vi "Page_Advanced_Initialize.vi"(6 "ctl references":T1, 8 "error in (no error)":errorcluster, 11 "AB_EXE in":refnum<class "AB_EXE.lvclass">) -> (0 "error out":errorcluster, 3 "AB_EXE out":refnum<class "AB_EXE.lvclass">)   [LabVIEW 2020, in "AB_EXE.lvclass"]
uses:
  <vilib>/AppBuilder/AB_Classes/EXE/AB_EXE.lvclass
  <resource>/Framework/Providers/Builds/AppBuilder/AB_UI_Page_Advanced_References.ctl
  <resource>/Framework/Providers/Common/provcom_StringGlobals.vi
  <vilib>/AppBuilder/AB_Classes/Application/AB_Application.lvclass
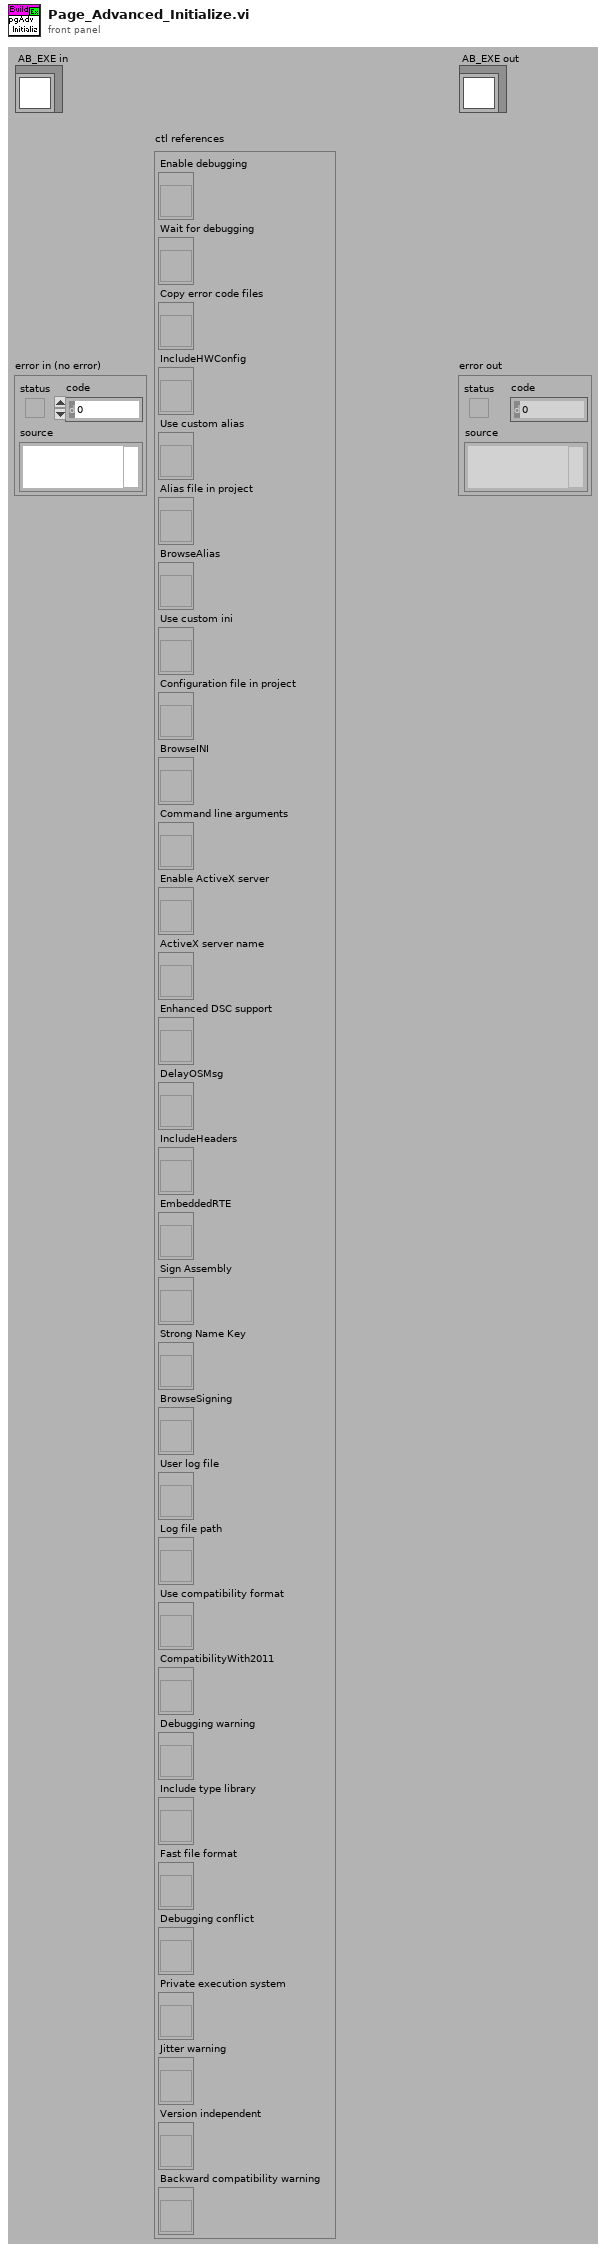
[diagram p1: front panel]
types:
  T1 = typedef "AB_UI_Page_Advanced_References.ctl" = cluster{"Enable debugging":refnum<vi>, "Wait for debugging":refnum<vi>, "Copy error code files":refnum<vi>, "IncludeHWConfig":refnum<vi>, "Use custom alias":refnum<vi>, "Alias file in project":refnum<vi>, "BrowseAlias":refnum<vi>, "Use custom ini":refnum<vi>, "Configuration file in project":refnum<vi>, "BrowseINI":refnum<vi>, "Command line arguments":refnum<vi>, "Enable ActiveX server":refnum<vi>, "ActiveX server name":refnum<vi>, "Enhanced DSC support":refnum<vi>, "DelayOSMsg":refnum<vi>, "IncludeHeaders":refnum<vi>, "EmbeddedRTE":refnum<vi>, "Sign Assembly":refnum<vi>, "Strong Name Key":refnum<vi>, "BrowseSigning":refnum<vi>, "User log file":refnum<vi>, "Log file path":refnum<vi>, "Use compatibility format":refnum<vi>, "CompatibilityWith2011":refnum<vi>, "Debugging warning":refnum<vi>, "Include type library":refnum<vi>, "Fast file format":refnum<vi>, "Debugging conflict":refnum<vi>, "Private execution system":refnum<vi>, "Jitter warning":refnum<vi>, "Version independent":refnum<vi>, "Backward compatibility warning":refnum<vi>}
  T2 = enum32{"invalid OS target", "Mac OS", "Windows 3.1", "Windows 95/NT", "Solaris 1", "Solaris 2", "HP-UX", "PowerMAX", "Linux", "Irix", "Rhapsody", "BeOS", "AIX", "OSF1", "VxWorks", "PharLap", "Carbon", "RTX", "Windows x64", "Linux x64", "Mac OS X x64"}
  T3 = typedef "LVRectTypeDef.ctl" = cluster{"Left":i16, "Top":i16, "Right":i16, "Bottom":i16}
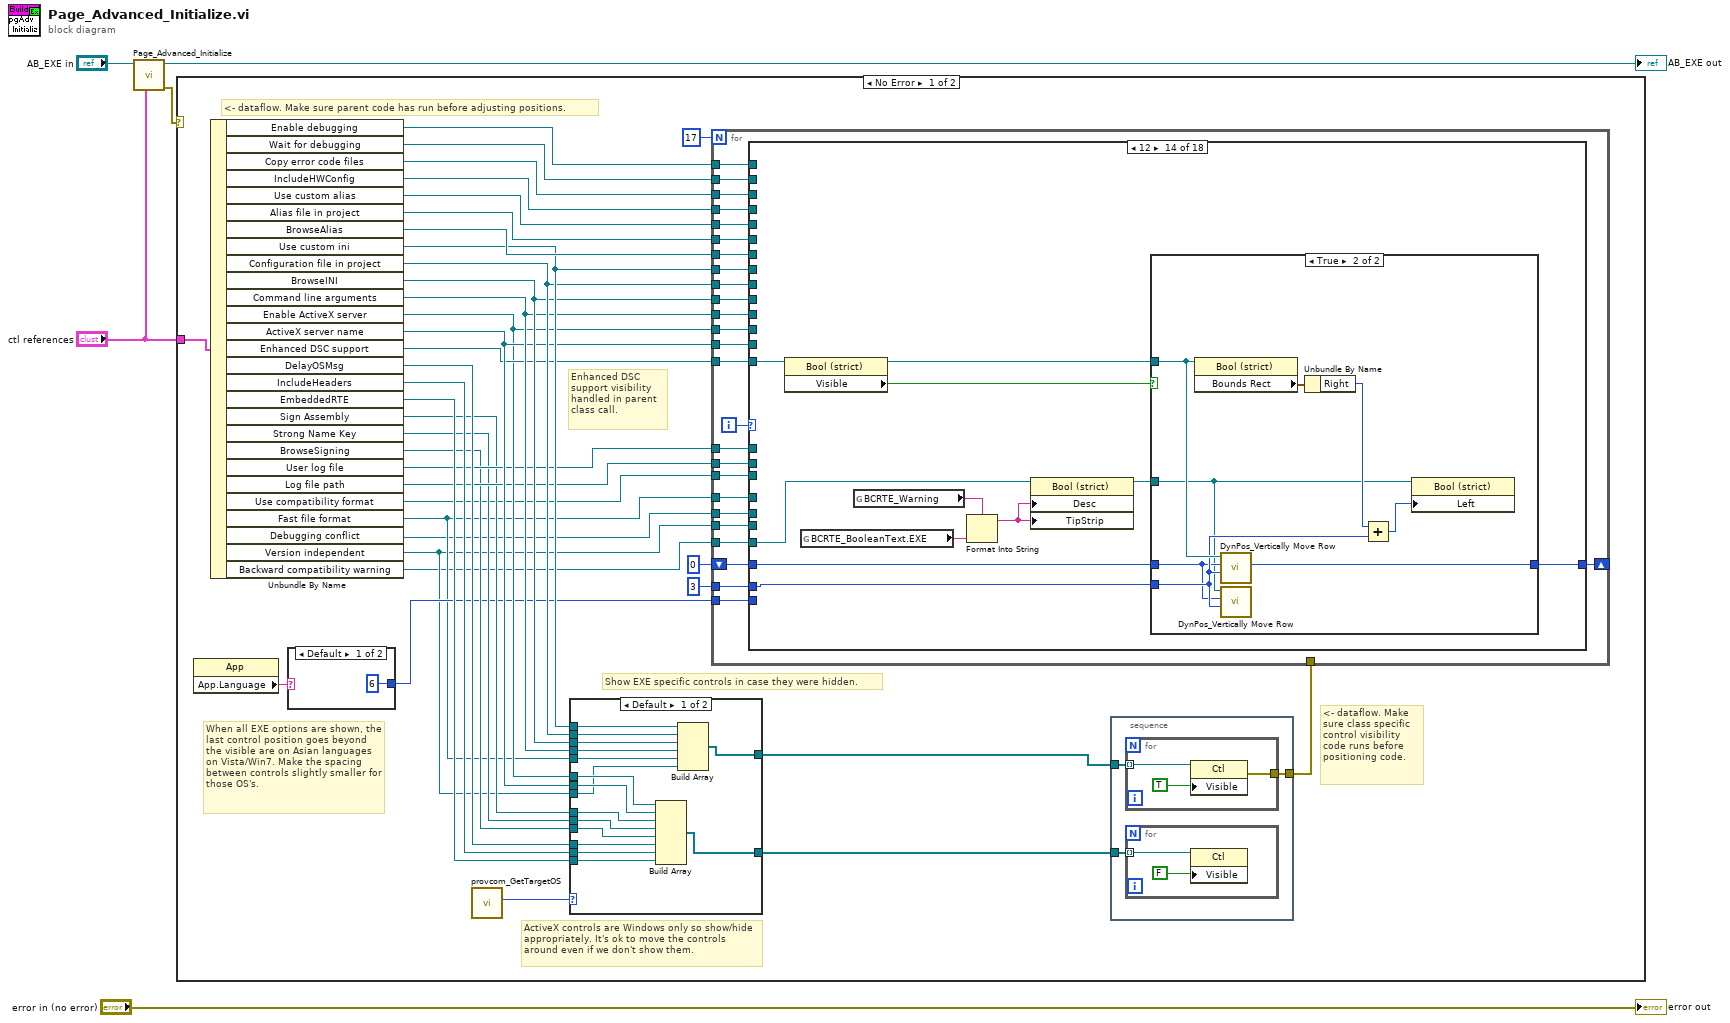
[diagram p0: block diagram]
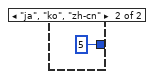
[diagram p2: hidden frame]
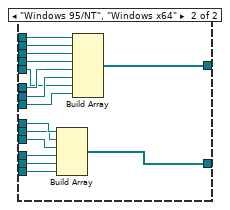
[diagram p3: hidden frame]
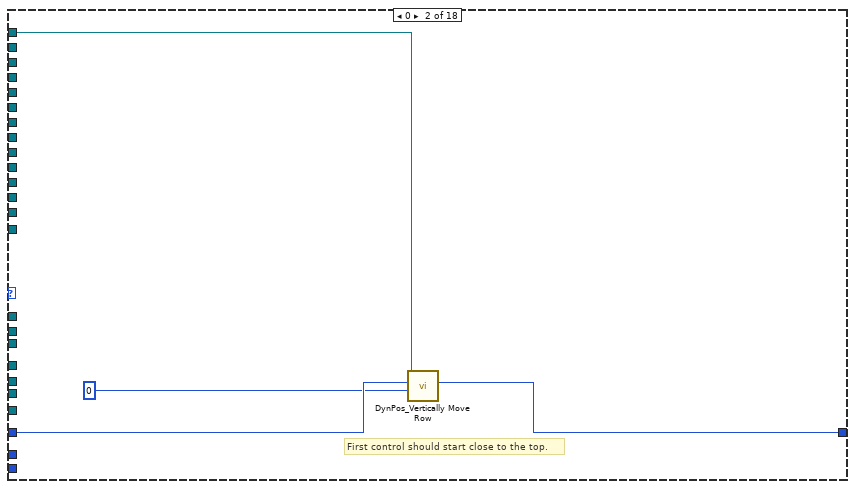
[diagram p5: hidden frame]
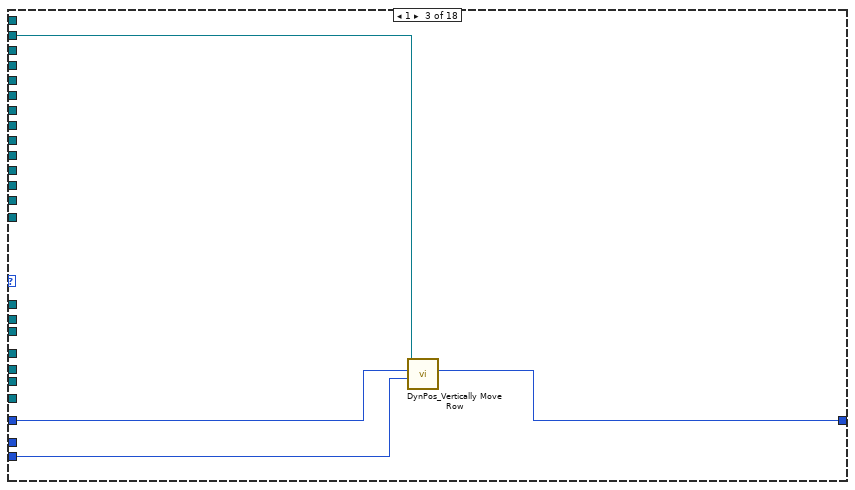
[diagram p6: hidden frame]
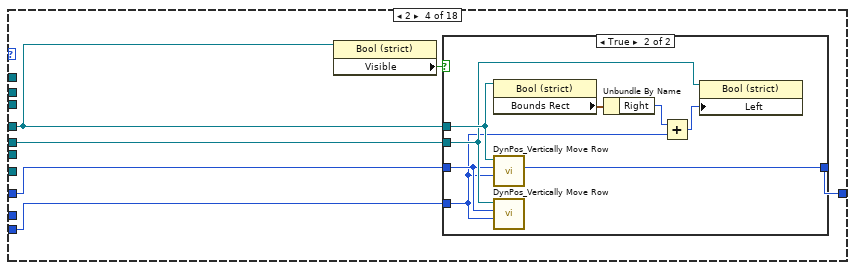
[diagram p7: hidden frame]
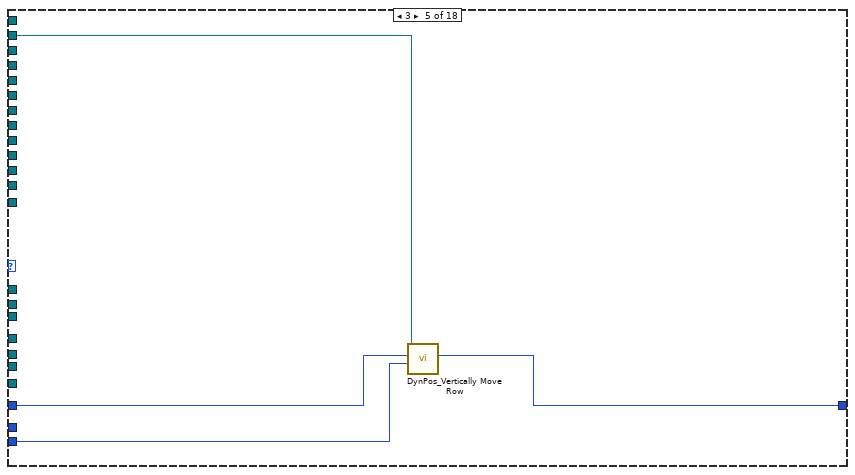
[diagram p9: hidden frame]
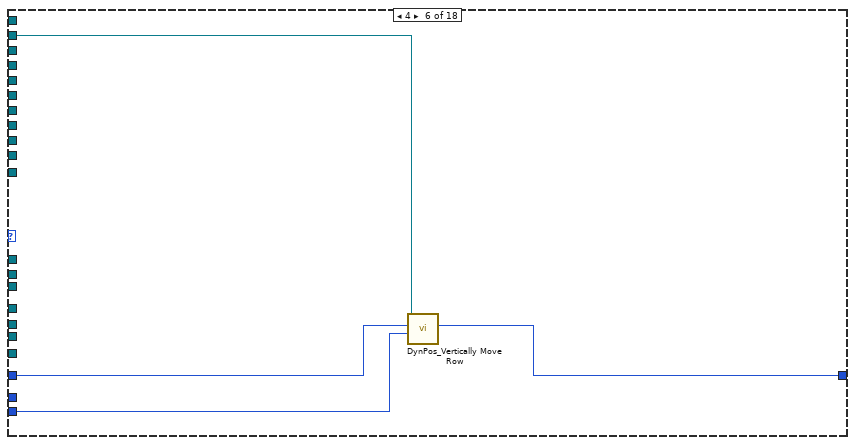
[diagram p10: hidden frame]
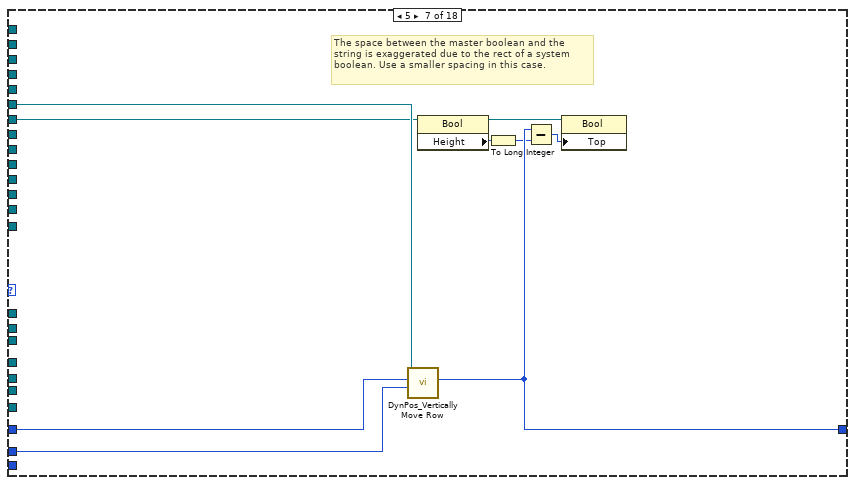
[diagram p11: hidden frame]
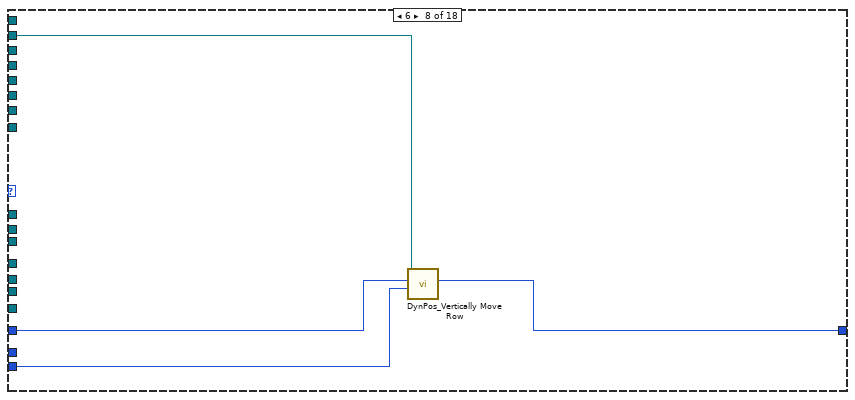
[diagram p12: hidden frame]
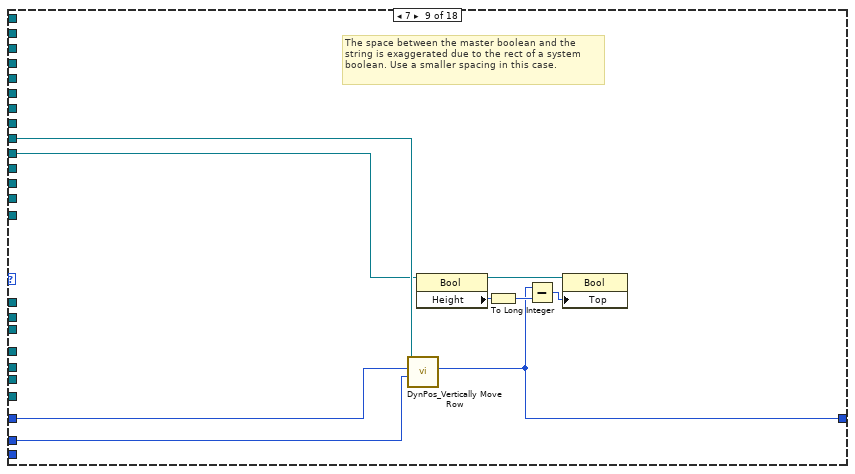
[diagram p13: hidden frame]
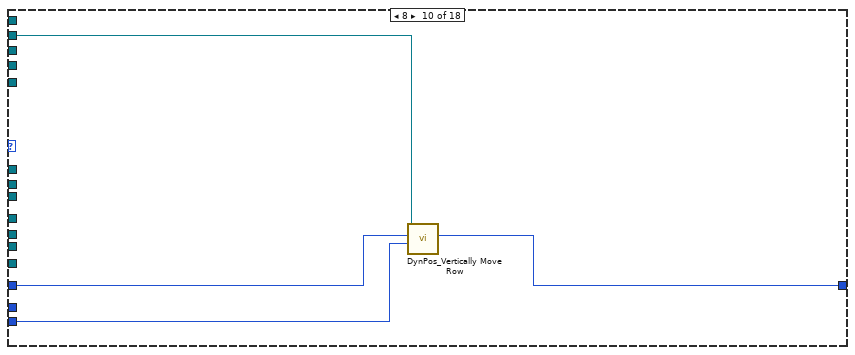
[diagram p14: hidden frame]
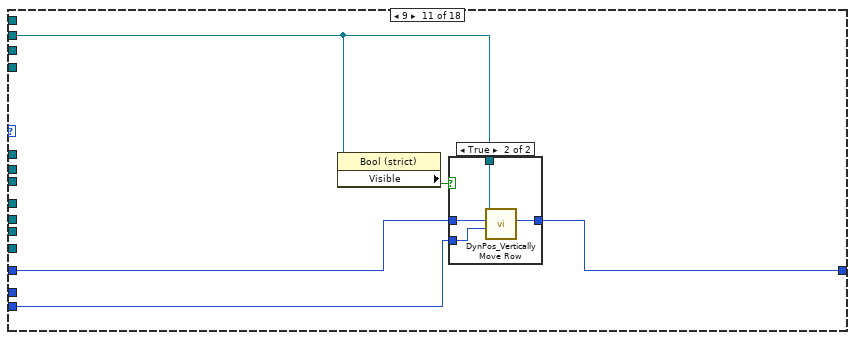
[diagram p15: hidden frame]
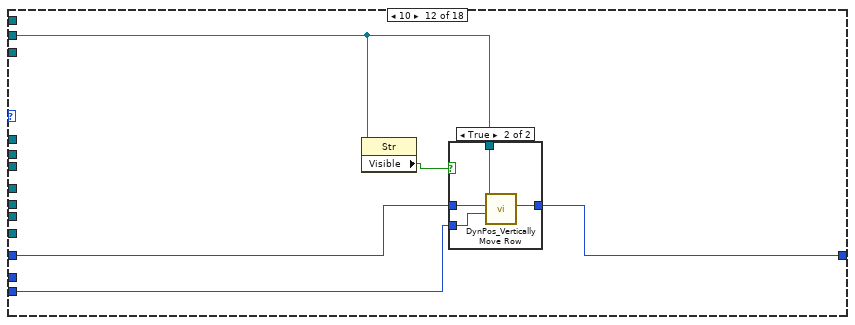
[diagram p17: hidden frame]
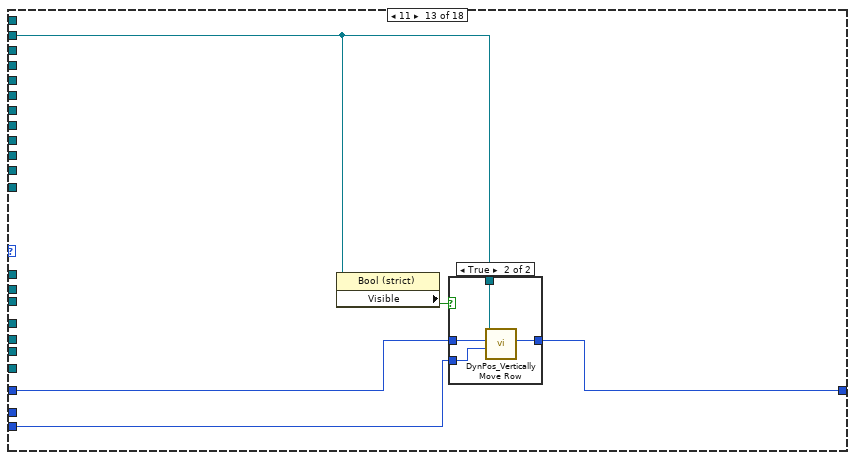
[diagram p19: hidden frame]
diagram:
  n1 = call-parent "Page_Advanced_Initialize.vi"("ctl references"="ctl references", "AB_Application in"="AB_EXE in") -> ("error out"=w1:errorcluster, "AB_Application out"=→"AB_EXE out":refnum<class "AB_EXE.lvclass">)  [unwired: 1 in, 7 out]
  n2 = case shown="No Error" w1 {
    tunnel: "ctl references" -> [w24 _]
    frame No Error {
      # "When all EXE options are shown, the last control position goes beyond the visible are on Asian languages on Vista/Win7. Make the spacing between controls slightly smaller for those OS's."
      # "<- dataflow. Make sure parent code has run before adjusting positions."
      # "<- dataflow. Make sure class specific control visibility code runs before positioning code."
      # "Enhanced DSC support visibility handled in parent class call."
      # "Show EXE specific controls in case they were hidden."
      # "ActiveX controls are Windows only so show/hide appropriately. It's ok to move the controls around even if we don't show them."
      n3 = property class="App"() -> ("App.Language"=w12:string)  [unwired: 2 in, 2 out]
      n4 = Unbundle By Name(w24) -> ("Enable debugging"=w39:refnum<vi>, "Wait for debugging"=w38:refnum<vi>, "Copy error code files"=w37:refnum<vi>, "IncludeHWConfig"=w36:refnum<vi>, "Use custom alias"=w35:refnum<vi>, "Alias file in project"=w34:refnum<vi>, "BrowseAlias"=w33:refnum<vi>, "Use custom ini"=w29:refnum<vi>, "Configuration file in project"=w28:refnum<vi>, "BrowseINI"=w27:refnum<vi>, "Command line arguments"=w26:refnum<vi>, "Enable ActiveX server"=w21:refnum<vi>, "ActiveX server name"=w23:refnum<vi>, "Enhanced DSC support"=w22:refnum<vi>, "DelayOSMsg"=w42:refnum<vi>, "IncludeHeaders"=w41:refnum<vi>, "EmbeddedRTE"=w40:refnum<vi>, "Sign Assembly"=w17:refnum<vi>, "Strong Name Key"=w16:refnum<vi>, "BrowseSigning"=w15:refnum<vi>, "User log file"=w18:refnum<vi>, "Log file path"=w19:refnum<vi>, "Use compatibility format"=w13:refnum<vi>, "Fast file format"=w9:refnum<vi>, "Debugging conflict"=w8:refnum<vi>, "Version independent"=w7:refnum<vi>, "Backward compatibility warning"=w6:refnum<vi>)
      n5 = case shown="Default" w12 {
        tunnel: [6 ("Bottom of last control") 5 ("Bottom of last control")] -> w11
        frame Default {
        }
        frame "ja", "ko", "zh-cn" {
        }
      }
      n6 = call <resource>:"provcom_GetTargetOS.vi"() -> ("App.TargetOS"=w20:T2)  [unwired: 11 out]
      n7 = case shown="Default" w20 {
        tunnel: w42 -> [w66 w84]
        tunnel: w41 -> [w67 w83]
        tunnel: w40 -> [w68 w82]
        tunnel: [w65 w81] -> w30
        tunnel: w23 -> [w58 w75]
        tunnel: w29 -> [w64 w80]
        tunnel: w28 -> [w63 w79]
        tunnel: w27 -> [w62 w78]
        tunnel: w26 -> [w61 w77]
        tunnel: [w60 w76] -> w25
        tunnel: w21 -> [w59 w74]
        tunnel: w17 -> [w57 w73]
        tunnel: w16 -> [w56 w72]
        tunnel: w15 -> [w55 w71]
        tunnel: w9 -> [w54 w70]
        tunnel: w7 -> [w53 w69]
        frame Default {
          n8 = Build Array(w59, w58, w57, w56, w55, w66, w67, w68) -> (w65:refnum<vi>[])
          n9 = Build Array(w64, w63, w62, w61, w54, w53) -> (w60:refnum<vi>[])
        }
        frame "Windows 95/NT", "Windows x64" {
          n10 = Build Array(w73, w72, w71, w84, w83, w82) -> (w81:refnum<vi>[])
          n11 = Build Array(w80, w79, w78, w77, w74, w75, w70, w69) -> (w76:refnum<vi>[])
        }
      }
      n12 = stacked-sequence {
        tunnel: w30 -> [w47]
        tunnel: w25 -> [w46]
        tunnel: [w45] -> w14
        frame #0 {
          n13 = for {
            tunnel: w46 -> [w50] mode=indexing
            tunnel: [w48] -> w45
            n14 = property class="Ctl"(reference=w50, "Visible"=TRUE) -> (error out=w48:errorcluster)  [unwired: 1 in, 1 out]
          }
          n15 = for {
            tunnel: w47 -> [w52] mode=indexing
            n16 = property class="Ctl"(reference=w52, "Visible"=FALSE) -> ()  [unwired: 1 in, 2 out]
          }
        }
      }
      n17 = for {
        N: 17 -> [_]
        tunnel: w39 -> [w109]
        tunnel: w38 -> [w108]
        tunnel: w37 -> [w107]
        tunnel: w36 -> [w106]
        tunnel: w35 -> [w105]
        tunnel: w34 -> [w104]
        tunnel: w33 -> [w103]
        tunnel: w29 -> [w102]
        tunnel: w28 -> [w101]
        shift-right: [w98] -> _
        shift-left: 0 ("Bottom of last control") -> [w100]
        tunnel: w11 -> [w99]
        tunnel: w27 -> [w97]
        tunnel: w26 -> [w96]
        tunnel: w21 -> [w95]
        tunnel: w23 -> [w94]
        tunnel: w22 -> [w93]
        tunnel: w19 -> [w92]
        tunnel: w18 -> [w91]
        tunnel: w14 -> [_]
        tunnel: w13 -> [w90]
        tunnel: 3 ("Bottom of last control") -> [w89]
        tunnel: w9 -> [w88]
        tunnel: w8 -> [w87]
        tunnel: w7 -> [w86]
        tunnel: w6 -> [w85]
        i -> [w110]
        n18 = case shown="12" w110 {
          tunnel: w109 -> [_ w114 _ _ _ _ _ _ _ _ _ _ _ _ _ _ _ _]
          tunnel: w108 -> [_ _ w116 _ _ _ _ _ _ _ _ _ _ _ _ _ _ _]
          tunnel: w107 -> [_ _ _ _ w135 _ _ _ _ _ _ _ _ _ _ _ _ _]
          tunnel: w106 -> [_ _ _ _ _ _ _ _ _ _ _ _ w190 _ _ _ _ _]
          tunnel: w105 -> [_ _ _ _ _ w139 _ _ _ _ _ _ _ _ _ _ _ _]
          tunnel: w104 -> [_ _ _ _ _ _ w150 _ _ _ _ _ _ _ _ _ _ _]
          tunnel: w103 -> [_ _ _ _ _ _ w149 _ _ _ _ _ _ _ _ _ _ _]
          tunnel: w102 -> [_ _ _ _ _ _ _ w152 _ _ _ _ _ _ _ _ _ _]
          tunnel: w101 -> [_ _ _ _ _ _ _ _ w163 _ _ _ _ _ _ _ _ _]
          tunnel: w100 -> [w111 w115 w119 w123 w138 w142 w151 w155 w164 w168 w172 w182 w193 w206 w222 w226 w230 w238]
          tunnel: w99 -> [_ _ w118 w122 w137 w141 _ w154 _ w167 w171 w181 w192 _ w221 w225 w229 w237]
          tunnel: [w111 w113 w117 w125 w136 w140 w145 w153 w158 w166 w170 w180 w191 w209 w220 w224 w228 w236] -> w98
          tunnel: w97 -> [_ _ _ _ _ _ _ _ w159 _ _ _ _ _ _ _ _ _]
          tunnel: w96 -> [_ _ _ _ _ _ _ _ _ w165 _ _ _ _ _ _ _ _]
          tunnel: w95 -> [_ _ _ _ _ _ _ _ _ _ w169 _ _ _ _ _ _ _]
          tunnel: w94 -> [_ _ _ _ _ _ _ _ _ _ _ w179 _ _ _ _ _ _]
          tunnel: w93 -> [_ _ _ _ _ _ _ _ _ _ _ _ _ w204 _ _ _ _]
          tunnel: w92 -> [_ _ _ _ _ _ _ _ _ _ _ _ _ _ _ w223 _ _]
          tunnel: w91 -> [_ _ _ _ _ _ _ _ _ _ _ _ _ _ w219 _ _ _]
          tunnel: w90 -> [_ _ _ _ _ _ _ _ _ _ _ _ _ _ _ _ w227 _]
          tunnel: w89 -> [_ _ _ _ _ _ w143 _ w156 _ _ _ _ w207 _ _ _ _]
          tunnel: w88 -> [_ _ _ w121 _ _ _ _ _ _ _ _ _ _ _ _ _ _]
          tunnel: w87 -> [_ _ _ w124 _ _ _ _ _ _ _ _ _ _ _ _ _ _]
          tunnel: w86 -> [_ _ _ _ _ _ _ _ _ _ _ _ _ _ _ _ _ w234]
          tunnel: w85 -> [_ _ _ _ _ _ _ _ _ _ _ _ _ w203 _ _ _ _]
          frame Default {
          }
          frame 0 {
            # "First control should start close to the top."
            n19 = call <vilib>:"DynPos_Vertically Move Row.vi"("Pixel separation (6)"=0, "Bottom of last control"=w115, "Control"=w114) -> ("Bottom pixel"=w113:i32)  [unwired: 1 in, 7 out]
          }
          frame 1 {
            n20 = call <vilib>:"DynPos_Vertically Move Row.vi"("Pixel separation (6)"=w118, "Bottom of last control"=w119, "Control"=w116) -> ("Bottom pixel"=w117:i32)  [unwired: 1 in, 7 out]
          }
          frame 2 {
            n21 = property class="Bool (strict)"(reference=w121) -> ("Visible"=w120:bool)  [unwired: 1 in, 2 out]
            n22 = case shown="True" w120 {
              tunnel: [w126 w134] -> w125
              tunnel: w121 -> [_ w130]
              tunnel: w124 -> [_ w129]
              tunnel: w123 -> [w126 w128]
              tunnel: w122 -> [_ w127]
              frame False {
              }
              frame True {
                n23 = property class="Bool (strict)"(reference=w130) -> ("Bounds Rect"=w133:T3)  [unwired: 1 in, 2 out]
                n24 = call <vilib>:"DynPos_Vertically Move Row.vi"("Pixel separation (6)"=w127, "Bottom of last control"=w128, "Control"=w130) -> ("Bottom pixel"=w134:i32)  [unwired: 1 in, 7 out]
                n25 = call <vilib>:"DynPos_Vertically Move Row.vi"("Pixel separation (6)"=w127, "Bottom of last control"=w128, "Control"=w129) -> ()  [unwired: 1 in, 8 out]
                n26 = Unbundle By Name(w133) -> ("Right"=w132:i16)
                n27 = Add(x=w132, y=w127) -> (x+y=w131:i32)
                n28 = property class="Bool (strict)"(reference=w129, "Left"=w131) -> ()  [unwired: 1 in, 2 out]
              }
            }
          }
          frame 3 {
            n29 = call <vilib>:"DynPos_Vertically Move Row.vi"("Pixel separation (6)"=w137, "Bottom of last control"=w138, "Control"=w135) -> ("Bottom pixel"=w136:i32)  [unwired: 1 in, 7 out]
          }
          frame 4 {
            n30 = call <vilib>:"DynPos_Vertically Move Row.vi"("Pixel separation (6)"=w141, "Bottom of last control"=w142, "Control"=w139) -> ("Bottom pixel"=w140:i32)  [unwired: 1 in, 7 out]
          }
          frame 5 {
            # "The space between the master boolean and the string is exaggerated due to the rect of a system boolean. Use a smaller spacing in this case."
            n31 = call <vilib>:"DynPos_Vertically Move Row.vi"("Pixel separation (6)"=w143, "Bottom of last control"=w151, "Control"=w150) -> ("Bottom pixel"=w145:i32)  [unwired: 1 in, 7 out]
            n32 = property class="Bool"(reference=w149) -> (reference out=w148:refnum<vi>, "Height"=w147:u32)  [unwired: 1 in, 1 out]
            n33 = To Long Integer(number=w147) -> (32bit integer=w144:i32)
            n34 = Subtract(x=w145, y=w144) -> (x-y=w146:i32)
            n35 = property class="Bool"(reference=w148, "Top"=w146) -> ()  [unwired: 1 in, 2 out]
          }
          frame 6 {
            n36 = call <vilib>:"DynPos_Vertically Move Row.vi"("Pixel separation (6)"=w154, "Bottom of last control"=w155, "Control"=w152) -> ("Bottom pixel"=w153:i32)  [unwired: 1 in, 7 out]
          }
          frame 7 {
            # "The space between the master boolean and the string is exaggerated due to the rect of a system boolean. Use a smaller spacing in this case."
            n37 = call <vilib>:"DynPos_Vertically Move Row.vi"("Pixel separation (6)"=w156, "Bottom of last control"=w164, "Control"=w163) -> ("Bottom pixel"=w158:i32)  [unwired: 1 in, 7 out]
            n38 = property class="Bool"(reference=w159) -> (reference out=w162:refnum<vi>, "Height"=w161:u32)  [unwired: 1 in, 1 out]
            n39 = To Long Integer(number=w161) -> (32bit integer=w160:i32)
            n40 = Subtract(x=w158, y=w160) -> (x-y=w157:i32)
            n41 = property class="Bool"(reference=w162, "Top"=w157) -> ()  [unwired: 1 in, 2 out]
          }
          frame 8 {
            n42 = call <vilib>:"DynPos_Vertically Move Row.vi"("Pixel separation (6)"=w167, "Bottom of last control"=w168, "Control"=w165) -> ("Bottom pixel"=w166:i32)  [unwired: 1 in, 7 out]
          }
          frame 9 {
            n43 = property class="Bool (strict)"(reference=w169) -> ("Visible"=w173:bool)  [unwired: 1 in, 2 out]
            n44 = case shown="True" w173 {
              tunnel: w172 -> [w174 w178]
              tunnel: w171 -> [_ w177]
              tunnel: [w174 w176] -> w170
              tunnel: w169 -> [_ w175]
              frame False {
              }
              frame True {
                n45 = call <vilib>:"DynPos_Vertically Move Row.vi"("Pixel separation (6)"=w177, "Bottom of last control"=w178, "Control"=w175) -> ("Bottom pixel"=w176:i32)  [unwired: 1 in, 7 out]
              }
            }
          }
          frame 10 {
            n46 = property class="Str"(reference=w179) -> ("Visible"=w183:bool)  [unwired: 1 in, 2 out]
            n47 = case shown="True" w183 {
              tunnel: w182 -> [w184 w188]
              tunnel: w181 -> [_ w187]
              tunnel: [w184 w186] -> w180
              tunnel: w179 -> [_ w185]
              frame False {
              }
              frame True {
                n48 = call <vilib>:"DynPos_Vertically Move Row.vi"("Pixel separation (6)"=w187, "Bottom of last control"=w188, "Control"=w185) -> ("Bottom pixel"=w186:i32)  [unwired: 1 in, 7 out]
              }
            }
          }
          frame 11 {
            n49 = property class="Bool (strict)"(reference=w190) -> ("Visible"=w189:bool)  [unwired: 1 in, 2 out]
            n50 = case shown="True" w189 {
              tunnel: w193 -> [w194 w198]
              tunnel: w192 -> [_ w197]
              tunnel: [w194 w196] -> w191
              tunnel: w190 -> [_ w195]
              frame False {
              }
              frame True {
                n51 = call <vilib>:"DynPos_Vertically Move Row.vi"("Pixel separation (6)"=w197, "Bottom of last control"=w198, "Control"=w195) -> ("Bottom pixel"=w196:i32)  [unwired: 1 in, 7 out]
              }
            }
          }
          frame 12 {
            n52 = property class="Bool (strict)"(reference=w204) -> (reference out=w205:refnum<vi>, "Visible"=w208:bool)  [unwired: 1 in, 1 out]
            n53 = global read "provcom_StringGlobals.vi" "BCRTE_BooleanText.EXE"() -> (w200:string)
            n54 = global read "provcom_StringGlobals.vi" "BCRTE_Warning"() -> (w201:string)
            n55 = Format Into String(format string=w201, w200) -> (resulting string=w199:string)  [unwired: 2 in, 1 out]
            n56 = property class="Bool (strict)"(reference=w203, "Desc"=w199, "TipStrip"=w199) -> (reference out=w202:refnum<vi>)  [unwired: 1 in, 1 out]
            n57 = case shown="True" w208 {
              tunnel: w206 -> [w210 w212]
              tunnel: w207 -> [_ w213]
              tunnel: [w210 w215] -> w209
              tunnel: w205 -> [_ w214]
              tunnel: w202 -> [_ w211]
              frame False {
              }
              frame True {
                n58 = property class="Bool (strict)"(reference=w214) -> ("Bounds Rect"=w218:T3)  [unwired: 1 in, 2 out]
                n59 = call <vilib>:"DynPos_Vertically Move Row.vi"("Pixel separation (6)"=w213, "Bottom of last control"=w212, "Control"=w214) -> ("Bottom pixel"=w215:i32)  [unwired: 1 in, 7 out]
                n60 = call <vilib>:"DynPos_Vertically Move Row.vi"("Pixel separation (6)"=w213, "Bottom of last control"=w212, "Control"=w211) -> ()  [unwired: 1 in, 8 out]
                n61 = Unbundle By Name(w218) -> ("Right"=w217:i16)
                n62 = Add(x=w217, y=w213) -> (x+y=w216:i32)
                n63 = property class="Bool (strict)"(reference=w211, "Left"=w216) -> ()  [unwired: 1 in, 2 out]
              }
            }
          }
          frame 13 {
            n64 = call <vilib>:"DynPos_Vertically Move Row.vi"("Pixel separation (6)"=w221, "Bottom of last control"=w222, "Control"=w219) -> ("Bottom pixel"=w220:i32)  [unwired: 1 in, 7 out]
          }
          frame 14 {
            n65 = call <vilib>:"DynPos_Vertically Move Row.vi"("Pixel separation (6)"=w225, "Bottom of last control"=w226, "Control"=w223) -> ("Bottom pixel"=w224:i32)  [unwired: 1 in, 7 out]
          }
          frame 15 {
            n66 = call <vilib>:"DynPos_Vertically Move Row.vi"("Pixel separation (6)"=w229, "Bottom of last control"=w230, "Control"=w227) -> ("Bottom pixel"=w228:i32)  [unwired: 1 in, 7 out]
          }
          frame 16 {
            n67 = global read "provcom_StringGlobals.vi" "BCRTE_BooleanText.EXE"() -> (w232:string)
            n68 = global read "provcom_StringGlobals.vi" "BCRTE_Description.EXE"() -> (w231:string)
            n69 = property class="Bool (strict)"(reference=w234, "BoolText.Text"=w232, "Desc"=w231) -> (reference out=w233:refnum<vi>, "Visible"=w235:bool)  [unwired: 1 in, 1 out]
            n70 = case shown="True" w235 {
              tunnel: w238 -> [w239 w243]
              tunnel: w237 -> [_ w242]
              tunnel: [w239 w241] -> w236
              tunnel: w233 -> [_ w240]
              frame False {
              }
              frame True {
                n71 = call <vilib>:"DynPos_Vertically Move Row.vi"("Pixel separation (6)"=w242, "Bottom of last control"=w243, "Control"=w240) -> ("Bottom pixel"=w241:i32)  [unwired: 1 in, 7 out]
              }
            }
          }
        }
      }
    }
    frame Error {
    }
  }
  "error out" <- "error in (no error)"
